vi "RT Main User StarStop.vi"() -> ()   [LabVIEW 2009]
doc: "This example shows how to use Simulation Module and Control Design Toolkit together and how to transfer the controller from Design to Simulation. It also uses the 3D Picture Control Toolkit to animate the system.\nThis example is derived from the Quanser (www.quanser.com) 3 DOF Helicopter academic experiment."
uses:
  MyGlobal.vi
  <vilib>/Simulation/Scripting/Companion Diagram/SimConfigNode/SimDog.xnode
  <vilib>/Simulation/Scripting/Companion Diagram/SimConfigNode/SimParams.ctl
  <vilib>/Simulation/Scripting/Companion Diagram/SimConfigNode/_simSolvers.ctl
  <vilib>/Simulation/Implementation/Shared/SIMSCR Execution Mode.ctl
  <vilib>/rvi/interface/nirviOpenFPGA/nirviOpenFPGA.xnode
  FPGA Bitfiles/sbRIOController.lv~4B_sbRIO-9631_FPGA Main.vi.lvbitx
  FPGA/FPGA Main.vi
  <vilib>/FPGAPlugInAG/sbRIO-9631/nirviIntfOpen_sbRIO-9631.vi
  <vilib>/rvi/interface/nirviReadWriteControl/nirviReadWriteControl.xnode
  <vilib>/Utility/error.llb/Error Cluster From Error Code.vi
  <vilib>/rvi/errors/niLvFpgaAdjustHostInterfaceError.vi
  <vilib>/rvi/interface/common/niFpgaNodeNameForErrorReporting.ctl
  <vilib>/rvi/errors/niLvFpgaWhatHappensToTopLevelVI.ctl
  Heli SubVIs/cdex_Position PID.vi
  Heli SubVIs/cdex_Pitch PID.vi
  Heli SubVIs/cdex_Elevation PID.vi
  <vilib>/Simulation/Implementation/Shared/SIM Bundle Sim Info.vi
  <vilib>/Simulation/Implementation/Shared/NILVSim_GetModelError.vi
  <vilib>/Simulation/Implementation/Shared/SIM Unbundle Sim Info.vi
  <vilib>/Platform/TimedLoop/XDataNode/XDataNode.xnode
  <vilib>/Platform/TimedLoop/XDataNode/loadlvalarms.vi
  <vilib>/Platform/TimedLoop/XDataNode/timing_clust.ctl
  <vilib>/Platform/TimedLoop/XDataNode/nitl_modes.ctl
  <vilib>/Platform/TimedLoop/XDataNode/wakeup.ctl
  <vilib>/Simulation/Implementation/Shared/NILVSim_Initialize.vi
  <vilib>/Simulation/Implementation/Shared/NILVSim_FinishedLate.vi
  <vilib>/Simulation/Implementation/Shared/NILVSim_Manager.vi
  <vilib>/Simulation/Scripting/Editor Utilities/SIM subVI tag data.ctl
  <vilib>/Simulation/Scripting/Editor Utilities/SIM subVI execution type.ctl
  Read Encoder Data Tester.vi
  <vilib>/Simulation/Implementation/Shared/SIM Fire Discrete SubVI.vi
  PWM to Set.vi
  <vilib>/Simulation/SignalArithmetic/SIMX Gain/SIMX Gain.xnode
  <vilib>/Simulation/SignalArithmetic/Implementation/NILVSim Gain.llb/SIM Gain (scalar).vi
  Set to PWM.vi
  <vilib>/Simulation/Utility/SIMX Halt/SIMX Halt.xnode
  <vilib>/Simulation/Utility/Implementation/SIM Halt.vi
  <vilib>/Simulation/Implementation/Shared/NILVSim_FinalizeModel.vi
  <vilib>/rvi/interface/nirviCloseFPGA/nirviCloseFPGA.xnode
  <vilib>/FPGAPlugInAG/sbRIO-9631/nirviIntfClose_sbRIO-9631.vi
  <vilib>/Simulation/Implementation/XNodeFramework/AbstractNodes/SimX_SubsystemNode/SimX_SubsystemNode.xnode
  NiRioSrv.dll
  <vilib>/userDefined/High Color/nirio_resource_hc.ctl
  <vilib>/Platform/TimedLoop/XDataNode/XDNodeRunTimeDep.lvlib
panel:
  in  "stop":bool
  out "error out":errorcluster
  in  "GO":bool
  in  "Clock Divider (ticks)":u16=1
  in  "PWM Period (ticks)":u32=100000
  in  "Position Angle Setpoint":dbl(knob) scale=-180.0..180.0
  in  "Elevation Setpoint":dbl(slide) scale=0.0..20.0 scale format="%.2f"
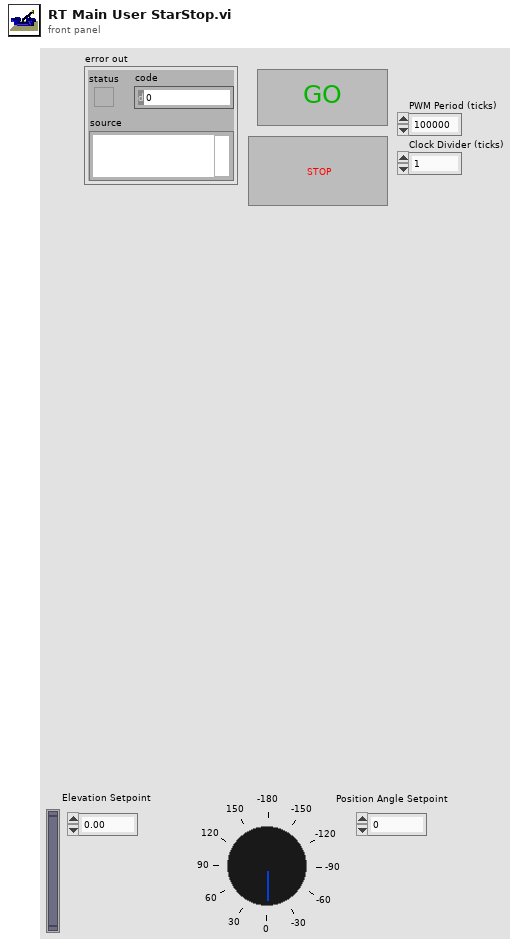
[diagram p1: front panel]
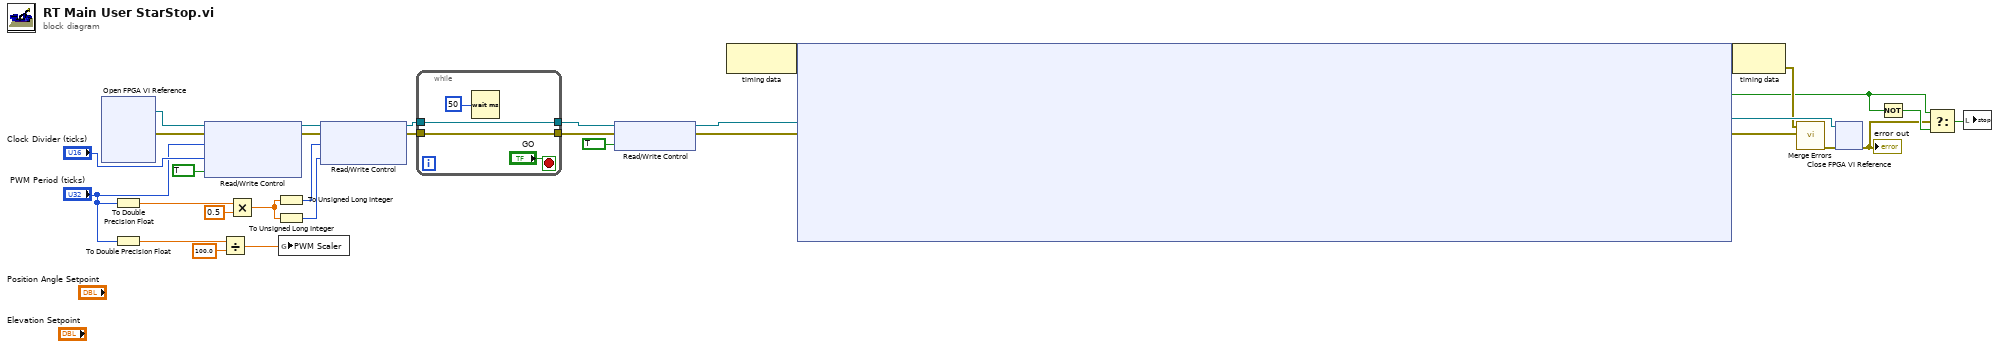
[diagram p0: block diagram]
diagram:
  n1 = xnode "Open FPGA VI Reference"() -> ("FPGA VI Reference Out"=w29:refnum<k20>, "error out"=w30:errorcluster)  [unwired: 2 in]
  n2 = To Double Precision Float(number="PWM Period (ticks)") -> (double precision float=w10:dbl)
  n3 = To Double Precision Float(number="PWM Period (ticks)") -> (double precision float=w7:dbl)
  n4 = xnode "Read/Write Control"("FPGA VI Reference In"=w29, "error in"=w30, "PWM Period (ticks)"="PWM Period (ticks)", "Clock Divider"="Clock Divider (ticks)", "ENC In Clock"=TRUE) -> ("FPGA VI Reference Out"=w19:refnum<k20>, "error out"=w20:errorcluster)
  n5 = Divide(x=w7, y=100.0) -> (x/y=w11:dbl)
  n6 = Multiply(x=w10, y=0.5) -> (x*y=w21:dbl)
  n7 = To Unsigned Long Integer(number=w21) -> (unsigned 32bit integer=w8:u32)
  n8 = To Unsigned Long Integer(number=w21) -> (unsigned 32bit integer=w9:u32)
  n9 = global write "MyGlobal.vi" "PWM Scaler"(w11) -> ()
  n10 = xnode "Read/Write Control"("FPGA VI Reference In"=w19, "error in"=w20, "Fan High Time 1"=w8, "Fan High Time 2"=w9) -> ("FPGA VI Reference Out"=w17:refnum<k20>, "error out"=w18:errorcluster)
  n11 = while {
    tunnel: w18 -> [w33]
    tunnel: w17 -> [w34]
    tunnel: [w34] -> w15
    tunnel: [w33] -> w16
    stop <- "GO" stop-if-true
    n12 = Wait (ms)(milliseconds to wait=u32 50) -> ()  [unwired: 1 out]
  }
  n13 = xnode "Read/Write Control"("FPGA VI Reference In"=w15, "error in"=w16, "Start Encoders"=TRUE) -> ("FPGA VI Reference Out"=w12:refnum<k20>, "error out"=w13:errorcluster)
  n14 = node-c288() -> (w2:variant)  [unwired: 1 in]
  n15 = node-c254 ("Simulation Loop")(w2, w13, w12) -> (w1:variant, w25:errorcluster, w27:refnum<k20>, w5:bool)
  n16 = node-c288(w1) -> (w26:errorcluster)
  n17 = call <vilib>:"Merge Errors.vi"("error in 2 (no error)"=w25, "error in 1 (no error)"=w26) -> ("error out"=w24:errorcluster)  [unwired: 5 in]
  n18 = xnode "Close FPGA VI Reference"("FPGA VI Reference In"=w27, "error in"=w24) -> ("error out"=w3:errorcluster)
  "error out" <- w3
  n19 = Not(x=w5) -> (.not. x?=w4:bool)
  n20 = Select(t=w5, s=w3, f=w4) -> (s? t:f=w6:bool)
  n21 = local write "stop"(w6) -> ()
